vi "Data.vi"() -> ()   [LabVIEW 2009]
panel:
  in  "Array":dbl[](array[numeric])
  out "data1":dbl[][](array[numeric])
  in  "wait":dbl
  in  "Data":u16[](array[numeric])
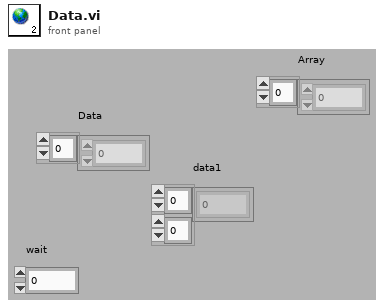
[diagram p1: front panel]
diagram:
